vi "Delete Templates in Oneof LVClasses.vi"(8 "error in (no error)":errorcluster, 11 "Library in":refnum<vi>) -> (0 "error out":errorcluster, 3 "Library out":refnum<vi>)   [LabVIEW 2019, in "gRPC Template Creation Utility.lvlib"]
uses:
  gRPC Template Creation Utility.lvlib
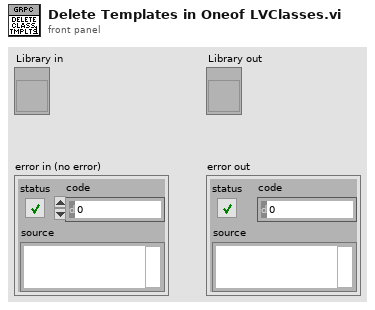
[diagram p1: front panel]
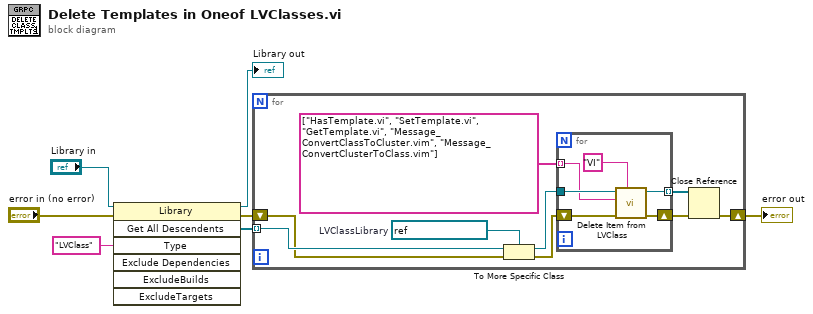
[diagram p0: block diagram]
diagram:
  n1 = invoke class="Library" method="Get All Descendents"(reference="Library in", error in="error in (no error)", "Type"="LVClass") -> (reference out=→"Library out":refnum<vi>, error out=w6:errorcluster, "All Descendents"=w5:refnum<vi>[])  [unwired: 4 in, 4 out]
  n2 = for {
    tunnel: w5 -> [w16] mode=indexing
    shift-right: [w8] -> w7
    shift-left: w6 -> [w11]
    w14 = refnum<vi> refnum  # LVClassLibrary
    n3 = To More Specific Class(target class=w14, reference=w16, error in=w11) -> (specific class reference=w15:refnum<vi>, error out=w12:errorcluster)
    n4 = for {
      tunnel: w15 -> [w22]
      tunnel: string[] ["HasTemplate.vi", "SetTemplate.vi", "GetTemplate.vi", "Message_ConvertClassToCluster.vim", "Message_ConvertClusterToClass.vim"] -> [w20] mode=indexing
      shift-right: [w18] -> w10
      shift-left: w12 -> [w19]
      tunnel: [w17] -> w9 mode=indexing
      n5 = call "Delete Item from LVClass.vi"("Item Type"="VI", "error in (no error)"=w19, "Item name"=w20, "LVClassLibrary in"=w22) -> ("error out"=w18:errorcluster, "LVClassLibrary out"=w17:refnum<vi>)  [unwired: 5 in, 1 out]
    }
    n6 = Close Reference(reference=w9, error in (no error)=w10) -> (error out=w8:errorcluster)
  }
  "error out" <- w7
